vi "Array Average.vi"(11 "Array In":dbl[](array[numeric])) -> (3 "Average out":dbl)   [LabVIEW 2014]
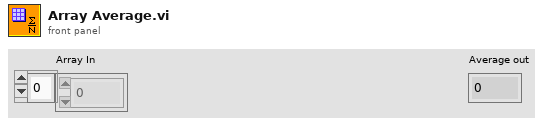
[diagram p1: front panel]
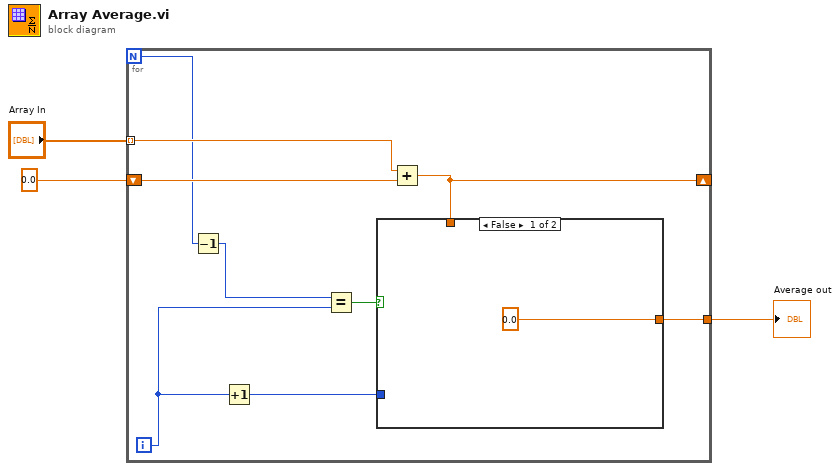
[diagram p0: block diagram]
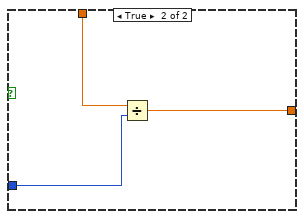
[diagram p2: hidden frame]
diagram:
  n1 = for {
    N -> [w10]
    tunnel: "Array In" -> [w12] mode=indexing
    shift-right: [w6] -> _
    shift-left: 0.0 -> [w11]
    tunnel: [w4] -> w1
    i -> [w8]
    n2 = Decrement(x=w10) -> (x-1=w9:i32)
    n3 = Increment(x=w8) -> (x+1=w5:i32)
    n4 = Equal?(x=w9, y=w8) -> (x = y?=w7:bool)
    n5 = Add(x=w12, y=w11) -> (x+y=w6:dbl)
    n6 = case shown="False" w7 {
      tunnel: w6 -> [_ w16]
      tunnel: w5 -> [_ w15]
      tunnel: [0.0 w14] -> w4
      frame False {
      }
      frame True {
        n7 = Divide(x=w16, y=w15) -> (x/y=w14:dbl)
      }
    }
  }
  "Average out" <- w1
